vi "Enum Data Patch.vi"(7 "Ref":variant, 8 "error in (no error)":errorcluster, 11 "data in":variant) -> (0 "error out":errorcluster, 3 "data out":variant)   [LabVIEW 2017]
doc: "Patches the string values of an enum carried in data in, using the enum type information in Ref, so an enum whose labels have changed still decodes correctly."
uses:
  <vilib>/Utility/Data Type/NI_Data Type.lvlib
  _openG/_reuse_openG.lvlib
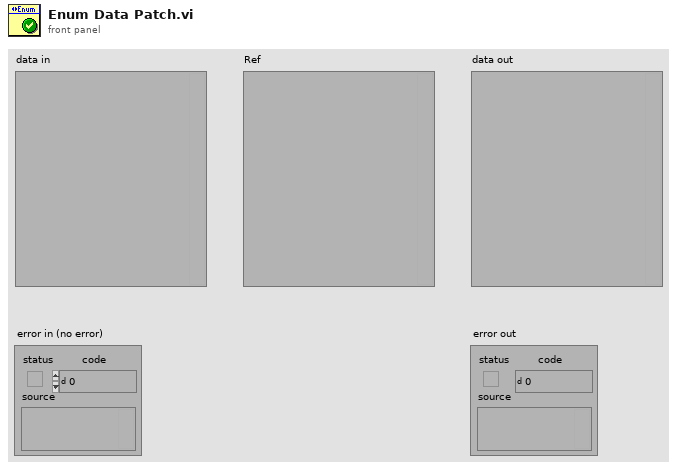
[diagram p1: front panel]
types:
  T1 = typedef "NI_Data Type.lvlib/Data Type.ctl" = enum8{"Invalid Type", "Void", "I8", "I16", "I32", "I64", "U8", "U16", "U32", "U64", "Single Float", "Double Float", "Extended Float", "Single Complex", "Double Complex", "Extended Complex", "Enum U8", "Enum U16", "Enum U32", "Enum U64", "Single Float With Unit", "Double Float With Unit", "Extended Float With Unit", "Single Complex with Unit", "Double Complex with Unit", "Extended Complex with Unit", "Boolean", "String", "Path", "Picture", "Tag", "Array", "Cluster", "Variant", "LV Variant", "Waveform", "Timestamp", "Digital Waveform", "Digital Data", "ExpressData", "Refnum", "External Data", "VI", "Poly VI", "LabVIEW Class Instance", "Fixed Point"}
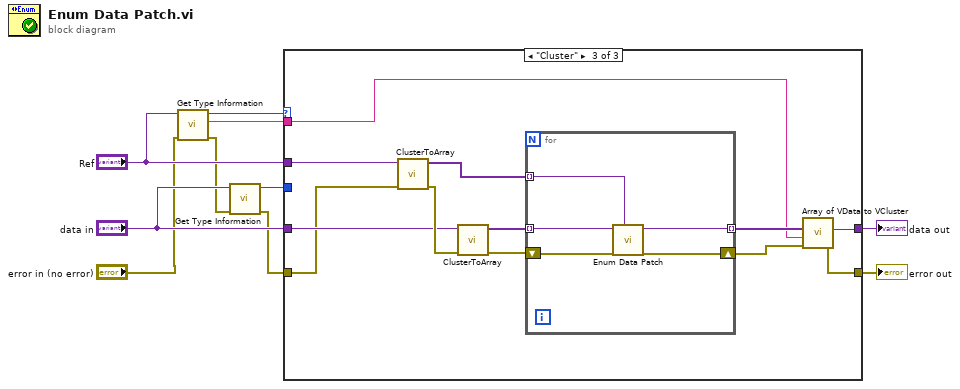
[diagram p0: block diagram]
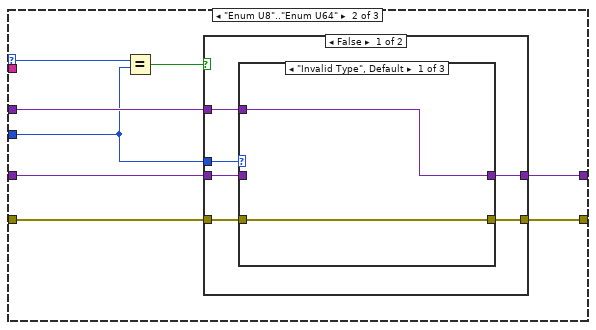
[diagram p3: hidden frame]
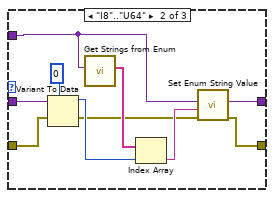
[diagram p4: hidden frame]
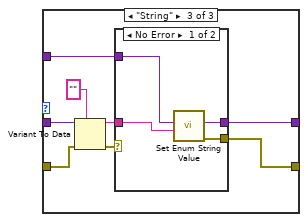
[diagram p5: hidden frame]
diagram:
  n1 = call <vilib>:"Get Type Information.vi"("error in (no error)"="error in (no error)", "Variant"="Ref") -> ("error out"=w5:errorcluster, "Name"=w2:string, "Type"=w7:T1)  [unwired: 5 in, 2 out]
  n2 = call <vilib>:"Get Type Information.vi"("error in (no error)"=w5, "Variant"="data in") -> ("error out"=w3:errorcluster, "Type"=w1:T1)  [unwired: 5 in, 3 out]
  n3 = case shown="\"Cluster\"" w7 {
    selector: w7 -> [_ w20 _]
    tunnel: [w12 w17 w65] -> w10
    tunnel: "data in" -> [w12 w14 w57]
    tunnel: w3 -> [w11 w15 w54]
    tunnel: [w11 w16 w60] -> w9
    tunnel: "Ref" -> [_ w18 w55]
    tunnel: w2 -> [_ _ w56]
    tunnel: w1 -> [_ w13 _]
    frame Default {
    }
    frame "Enum U8".."Enum U64" {
      n4 = Equal?(x=w20, y=w13) -> (x = y?=w19:bool)
      n5 = case shown="False" w19 {
        tunnel: w18 -> [w25 _]
        tunnel: [w23 w52] -> w17
        tunnel: [w22 w53] -> w16
        tunnel: w15 -> [w21 w53]
        tunnel: w14 -> [w24 w52]
        tunnel: w13 -> [w26 _]
        frame False {
          n6 = case shown="\"Invalid Type\", Default" w26 {
            tunnel: w25 -> [w28 w36 w45]
            tunnel: w24 -> [_ w38 w44]
            tunnel: [w28 w32 w46] -> w23
            tunnel: [w27 w30 w41] -> w22
            tunnel: w21 -> [w27 w29 w40]
            frame "Invalid Type", Default {
            }
            frame "I8".."U64" {
              n7 = Variant To Data(error in=w29, type=i64 0, Variant=w38) -> (data=w34:i64, error out=w31:errorcluster)
              n8 = call "Get Strings from Enum.vi"("Enum"=w36) -> ("Enum Strings"=w35:string[])  [unwired: 7 in, 3 out]
              n9 = Index Array(array=w35, index=w34) -> (element=w33:string)
              n10 = call "Set Enum String Value.vi"("error in (no error)"=w31, "String Value"=w33, "Default Enum Value"=w36) -> ("error out"=w30:errorcluster, "Enum"=w32:variant)  [unwired: 7 in]
            }
            frame "String" {
              n11 = Variant To Data(error in=w40, type="", Variant=w44) -> (data=w42:string, error out=w39:errorcluster)
              n12 = case shown="No Error" w39 {
                tunnel: [w50 w51] -> w46
                tunnel: w45 -> [w49 w51]
                tunnel: w42 -> [w48 _]
                tunnel: [w47 _] -> w41
                frame No Error {
                  n13 = call "Set Enum String Value.vi"("String Value"=w48, "Default Enum Value"=w49) -> ("error out"=w47:errorcluster, "Enum"=w50:variant)  [unwired: 8 in]
                }
                frame Error {
                }
              }
            }
          }
        }
        frame True {
        }
      }
    }
    frame "Cluster" {
      n14 = call "ClusterToArray.vi"("Error in"=w54, "Cluster"=w55) -> ("Error out"=w58:errorcluster, "Array"=w59:variant[])  [unwired: 8 in]
      n15 = call "ClusterToArray.vi"("Error in"=w58, "Cluster"=w57) -> ("Error out"=w62:errorcluster, "Array"=w64:variant[])  [unwired: 8 in]
      n16 = for {
        tunnel: w64 -> [w70] mode=indexing
        tunnel: [w69] -> w63 mode=indexing
        shift-right: [w67] -> w61
        shift-left: w62 -> [w68]
        tunnel: w59 -> [w66] mode=indexing
        n17 = call "Enum Data Patch.vi"("Ref"=w66, "error in (no error)"=w68, "data in"=w70) -> ("error out"=w67:errorcluster, "data out"=w69:variant)  [unwired: 7 in]
      }
      n18 = call "Array of VData to VCluster.vi"("error in (no error)"=w61, "Cluster Name"=w56, "Array"=w63) -> ("error out"=w60:errorcluster, "VCluster"=w65:variant)  [unwired: 7 in]
    }
  }
  "data out" <- w10
  "error out" <- w9
